vi "SDKSID4_Open SID4.vi"(4 "Error code in":errorcluster, 7 "User profile location":path) -> (0 "Error code out":errorcluster, 3 "SDKSID4 sessionID":T1)   [LabVIEW 2013]
doc: "This VI opens loads a new configuration file (user profile) in memory. It replaces the one already in memory. The inputs are the file path to the desired user profile and the file name of the mirror descriptor (located in the Mirror folder). If nothing is connected, the program loads the last ones previously loaded. The function outputs a unique reference ID that should be used as an input for all the other SID4 control functions."
uses:
  Refnum SDKSID4 session.ctl
  SID4_SDK.dll
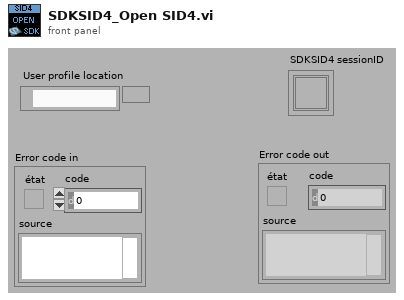
[diagram p1: front panel]
types:
  T1 = typedef "Refnum SDKSID4 session.ctl" = refnum<k1>
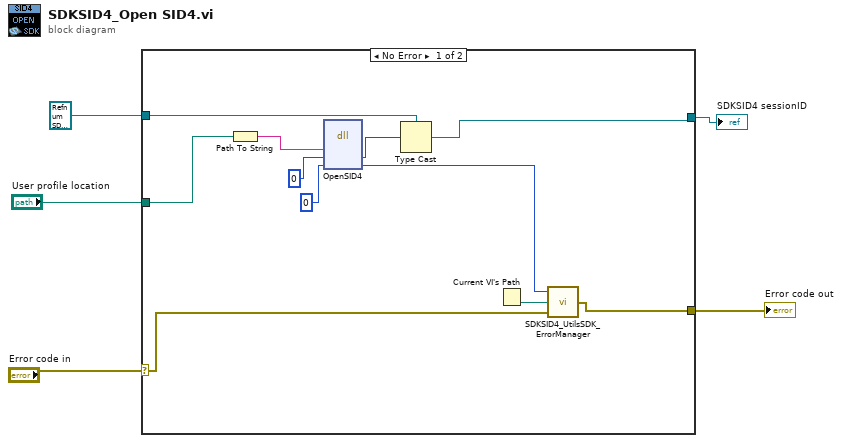
[diagram p0: block diagram]
diagram:
  n1 = case shown="No Error" "Error code in" {
    selector: "Error code in" -> [w10 w17]
    tunnel: [w15 w18] -> w5
    tunnel: T1 refnum ("SDKOASys session refnum") -> [w14 w18]
    tunnel: "User profile location" -> [w13 _]
    tunnel: [w11 w17] -> w1
    frame No Error {
      n2 = Path To String(path=w13) -> (string=w16:string)
      n3 = dll-call lib="C:/Program Files/SID4_SDK/DLL SDK/BIN/SID4_SDK.dll" fn="OpenSID4"("UserProfileLocation"=w16, "SessionID"=u32 0, "ErrorCode"=0) -> ("SessionID"=w6:u32, "ErrorCode"=w7:i32)  [unwired: 5 in, 2 out]
      n4 = Type Cast(type=w14, x=w6) -> (*(type *) &x=w15:T1)
      n5 = Current VI's Path() -> (path=w12:path)
      n6 = call "SDKSID4_UtilsSDK_ErrorManager.vi"("error IN"=w10, "VI PathFile"=w12, "ErrorCode"=w7) -> ("error OUT"=w11:errorcluster)
    }
    frame Error {
    }
  }
  "Error code out" <- w1
  "SDKSID4 sessionID" <- w5
